vi "ShoulderExecuteLogic.vi"(8 "error in (no error)":errorcluster, 10 "LowLimitSwitch":bool, 11 "PositionDeg":dbl) -> (0 "error out":errorcluster, 3 "MotorDemand":dbl)   [LabVIEW 2023]
doc: "Arm Execute for 2024 robot"
uses:
  ShoulderGetSetpointEnum.ctl
  <vilib>/Rock Robotics/WPI/ThirdParty/JAS_Junk/TrajLib/VI/BoolCmd_Recv_Internal.vi
  <vilib>/Rock Robotics/WPI/ThirdParty/JAS_Junk/TrajLib/VI/BoolCmd_ObtainQueue.vi
  Elevator/ElevatorGlobal.vi
  <vilib>/Rock Robotics/WPI/ThirdParty/JAS_Junk/TrajLib/Trajectory_Library.lvlib
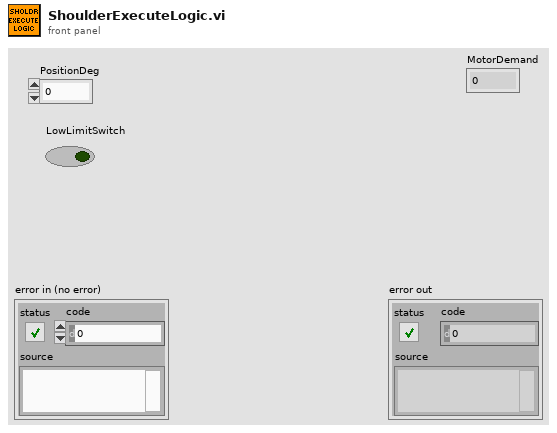
[diagram p1: front panel]
types:
  T1 = typedef "ShoulderGetSetpointEnum.ctl" = enum16{"ShoulderRest", "ShoulderSpeaker", "ShoulderAmp"}
  T2 = typedef "Trajectory_Library.lvlib/PosCtrl_Tuning_Type.ctl" = cluster{"Slope":dbl, "Offset":dbl, "Error Deadband":dbl, "At Reference Count":i32, "Negate Output":bool, "Max Allowd Position":dbl, "Min Allowd Position":dbl}
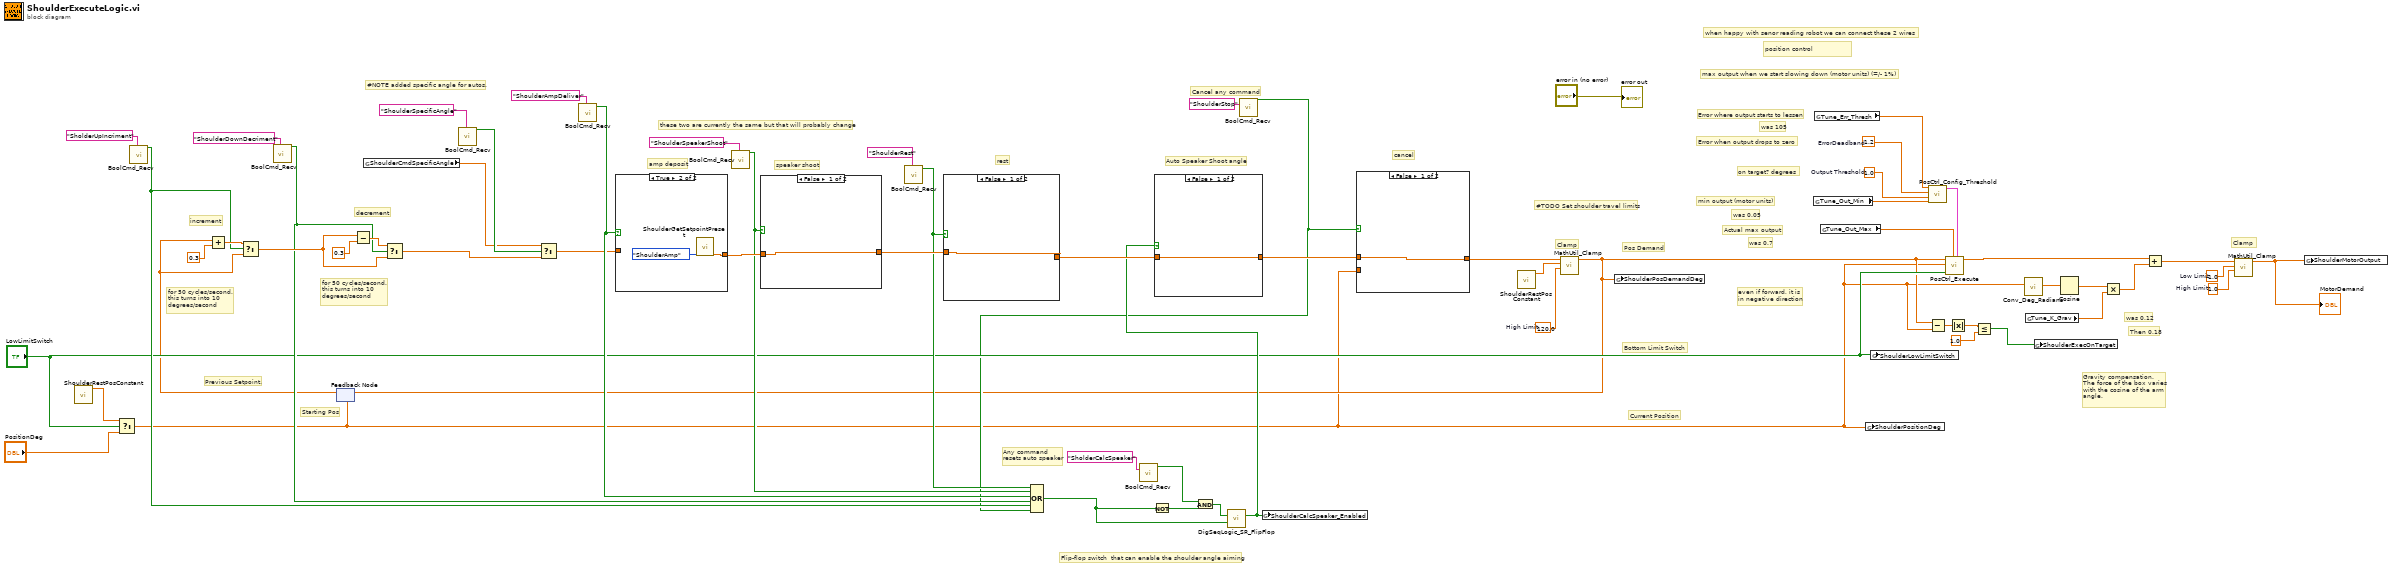
[diagram p0: block diagram]
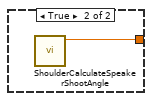
[diagram p2: hidden frame]
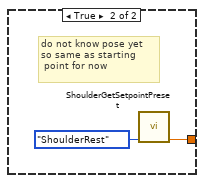
[diagram p4: hidden frame]
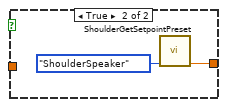
[diagram p5: hidden frame]
diagram:
  w40 = 120.0  # High Limit
  w46 = 1.0  # High Limit
  w45 = -1.0  # Low Limit
  w60 = 1.2  # ErrorDeadband
  w59 = 1.0  # Output Threshold
  # "#NOTE added specific angle for autos."
  # "was 0.05"
  # "was 0.7"
  # "Actual max output"
  # "Then 0.18"
  # "was 0.12"
  # "Previous Setpoint."
  # "Current Position"
  # "Bottom Limit Switch"
  # "Starting Pos"
  # "#TODO Set shoulder travel limits"
  # "Auto Speaker Shoot angle"
  # "Any command\nresets auto speaker"
  # "for 50 cycles/second.\nthis turns into 10 \ndegrees/second"
  # "for 50 cycles/second.\nthis turns into 10 \ndegrees/second"
  # "increment"
  # "Flip-flop switch  that can enable the shoulder angle aiming"
  # "Pos Demand"
  # "Clamp"
  # "was 105"
  # "Gravity compensation.\nThe force of the box varies\nwith the cosine of the arm\nangle."
  # "even if forward, it is \nin negative direction"
  # "these two are currently the same but that will probably change"
  # "Cancel any command"
  # "cancel"
  # "rest"
  # "speaker shoot"
  # "Clamp"
  # "amp deposit"
  # "decrement"
  # "when happy with senor reading robot we can connect these 2 wires"
  # "min output (motor units)"
  # "max output when we start slowing down (motor units) (=/- 1%)"
  # "on target? degrees"
  # "Error when output drops to zero"
  # "position control"
  # "Error where output starts to lessen"
  n1 = call "ShoulderRestPosConstant.vi"() -> ("RestPosition"=w7:dbl)  [unwired: 11 in]
  n2 = Select(t=w7, s="LowLimitSwitch", f="PositionDeg") -> (s? t:f=w17:dbl)
  n3 = call <vilib>:"BoolCmd_Recv.vi"("Command Name"="SholderUpIncriment") -> ("New Request"=w27:bool)  [unwired: 9 in, 1 out]
  n4 = call <vilib>:"BoolCmd_Recv.vi"("Command Name"="ShoulderDownDecriment") -> ("New Request"=w28:bool)  [unwired: 9 in, 1 out]
  n5 = feedback #1(w17) -> (w6:dbl)
  n6 = Add(x=w6, y=0.3) -> (x+y=w37:dbl)
  n7 = Select(t=w37, s=w27, f=w6) -> (s? t:f=w36:dbl)
  n8 = Subtract(x=w36, y=0.3) -> (x-y=w34:dbl)
  n9 = global read "ElevatorGlobal.vi" "ShoulderCmdSpecificAngle"() -> (w1:dbl)
  n10 = Select(t=w34, s=w28, f=w36) -> (s? t:f=w3:dbl)
  n11 = call <vilib>:"BoolCmd_Recv.vi"("Command Name"="ShoulderSpecificAngle") -> ("New Request"=w2:bool)  [unwired: 9 in, 1 out]
  n12 = Select(t=w1, s=w2, f=w3) -> (s? t:f=w4:dbl)
  n13 = call <vilib>:"BoolCmd_Recv.vi"("Command Name"="ShoulderAmpDeliver") -> ("New Request"=w29:bool)  [unwired: 9 in, 1 out]
  n14 = case shown="True" w29 {
    tunnel: w4 -> [w62 _]
    tunnel: [w62 w63] -> w58
    frame False {
    }
    frame True {
      n15 = call "ShoulderGetSetpointPreset.vi"("SholdrSetpoints"=ShoulderGetSetpointEnum."ShoulderAmp" ("ArmSetpoints")) -> ("Setpoint"=w63:dbl)  [unwired: 10 in]
    }
  }
  n16 = call <vilib>:"BoolCmd_Recv.vi"("Command Name"="ShoulderSpeakerShoot") -> ("New Request"=w30:bool)  [unwired: 9 in, 1 out]
  n17 = case shown="False" w30 {
    tunnel: w58 -> [w65 _]
    tunnel: [w65 w67] -> w39
    frame False {
    }
    frame True {
      n18 = call "ShoulderGetSetpointPreset.vi"("SholdrSetpoints"=ShoulderGetSetpointEnum."ShoulderSpeaker") -> ("Setpoint"=w67:dbl)  [unwired: 10 in]
    }
  }
  n19 = call <vilib>:"BoolCmd_Recv.vi"("Command Name"="ShoulderRest") -> ("New Request"=w31:bool)  [unwired: 9 in, 1 out]
  n20 = case shown="False" w31 {
    tunnel: w39 -> [w68 _]
    tunnel: [w68 w70] -> w33
    frame False {
    }
    frame True {
      # "do not know pose yet \nso same as starting\n point for now"
      n21 = call "ShoulderGetSetpointPreset.vi"("SholdrSetpoints"=ShoulderGetSetpointEnum."ShoulderRest") -> ("Setpoint"=w70:dbl)  [unwired: 10 in]
    }
  }
  n22 = call <vilib>:"BoolCmd_Recv.vi"("Command Name"="SholderCalcSpeaker") -> ("New Request"=w32:bool)  [unwired: 9 in, 1 out]
  n23 = call <vilib>:"BoolCmd_Recv.vi"("Command Name"="ShoulderStop") -> ("New Request"=w19:bool)  [unwired: 9 in, 1 out]
  n24 = Compound Arithmetic op=OR(w31, w30, w29, w28, w27, w19) -> (w26:bool)
  n25 = Not(x=w26) -> (.not. x?=w42:bool)
  n26 = And(x=w32, y=w42) -> (x .and. y?=w41:bool)
  n27 = call <vilib>:"DigSeqLogic_SR_FlipFlop.vi"("Set"=w41, "Reset"=w26) -> ("Output"=w24:bool)  [unwired: 12 in, 1 out]
  n28 = case shown="False" w24 {
    tunnel: w33 -> [w71 _]
    tunnel: [w71 w72] -> w25
    frame False {
    }
    frame True {
      n29 = call "ShoulderCalculateSpeakerShootAngle.vi"() -> ("ShoulderDesiredAngle (degrees)"=w72:dbl)  [unwired: 11 in]
    }
  }
  n30 = global write "ElevatorGlobal.vi" "ShoulderCalcSpeaker_Enabled"(w24) -> ()
  n31 = case shown="False" w19 {
    tunnel: w25 -> [w73 _]
    tunnel: [w73 w74] -> w22
    tunnel: w17 -> [_ w74]
    frame False {
    }
    frame True {
      # "takes get sensor pose pose"
    }
  }
  n32 = call "ShoulderRestPosConstant.vi"() -> ("RestPosition"=w8:dbl)  [unwired: 11 in]
  n33 = call <vilib>:"MathUtil_Clamp.vi"("High Limit"=w40, "Low Limit"=w8, "Value"=w22) -> ("Result"=w18:dbl)  [unwired: 8 in]
  n34 = feedback-in #1(w18) -> ()
  n35 = global write "ElevatorGlobal.vi" "ShoulderPosDemandDeg"(w18) -> ()
  n36 = global read "ElevatorGlobal.vi" "Tune_Out_Min"() -> (w10:dbl)
  n37 = global read "ElevatorGlobal.vi" "Tune_Err_Thresh"() -> (w9:dbl)
  n38 = global read "ElevatorGlobal.vi" "Tune_Out_Max"() -> (w11:dbl)
  n39 = global write "ElevatorGlobal.vi" "ShoulderPositionDeg"(w17) -> ()
  n40 = global write "ElevatorGlobal.vi" "ShoulderLowLimitSwitch"("LowLimitSwitch") -> ()
  n41 = call <vilib>:"PosCtrl_Config_Threshold.vi"("Output Deadband"=w10, "Output Threshold"=w59, "ErrorDeadband"=w60, "ErrorThreshold"=w9) -> ("PosCtrl_Config_Params"=w61:T2)  [unwired: 7 in]
  n42 = Subtract(x=w18, y=w17) -> (x-y=w16:dbl)
  n43 = call <vilib>:"PosCtrl_Execute.vi"("PosCtrl_Config_Params"=w61, "MaxOutput"=w11, "Rev Limit Switch"="LowLimitSwitch", "CurrentPosition"=w17, "TargetPosition"=w18) -> ("Output"=w50:dbl)  [unwired: 4 in, 2 out]
  n44 = Absolute Value(x=w16) -> (abs(x)=w15:dbl)
  n45 = Less Or Equal?(x=w15, y=1.0) -> (x <= y?=w13:bool)
  n46 = call <vilib>:"Conv_Deg_Radians.vi"("Degress"=w17) -> ("Radians"=w47:dbl)  [unwired: 10 in]
  n47 = global read "ElevatorGlobal.vi" "Tune_K_Grav"() -> (w12:dbl)
  n48 = global write "ElevatorGlobal.vi" "ShoulderExecOnTarget"(w13) -> ()
  n49 = Cosine(x=w47) -> (cos(x)=w48:dbl)
  n50 = Multiply(x=w48, y=w12) -> (x*y=w49:dbl)
  n51 = Add(x=w50, y=w49) -> (x+y=w44:dbl)
  n52 = call <vilib>:"MathUtil_Clamp.vi"("High Limit"=w46, "Low Limit"=w45, "Value"=w44) -> ("Result"=w20:dbl)  [unwired: 8 in]
  "MotorDemand" <- w20
  n53 = global write "ElevatorGlobal.vi" "ShoulderMotorOutput"(w20) -> ()
  "error out" <- "error in (no error)"
